vi "Path_to_Array_Of_Filepaths.vi"(4 "length":i32=1, 6 "offset (for subset of folder)":i32, 8 "error in (no error)":errorcluster, 11 "File or Folder Path":path=path "C:/") -> (0 "error out":errorcluster, 1 "pattern":string="*.dat", 3 "array of files":path[](array[path]))   [LabVIEW 2016]
uses:
  <userlib>/LevyLab/LV to ITX/LVtoITX.lvclass
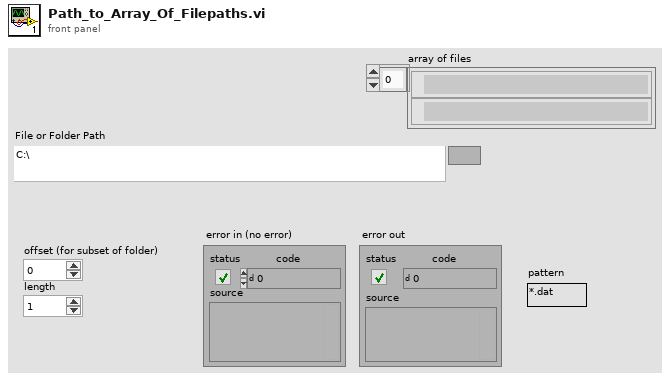
[diagram p1: front panel]
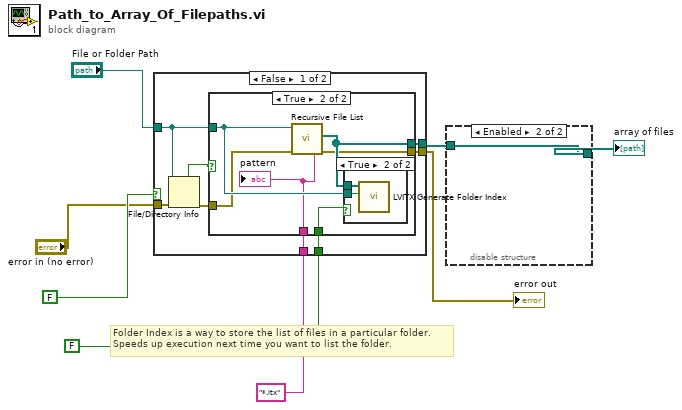
[diagram p0: block diagram]
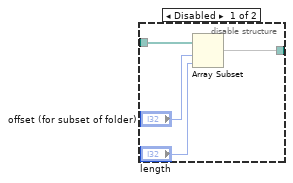
[diagram p2: hidden frame]
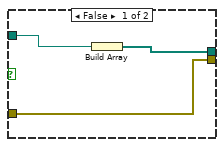
[diagram p3: hidden frame]
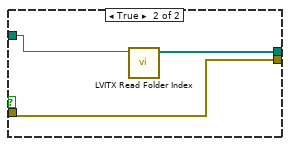
[diagram p5: hidden frame]
diagram:
  # "Folder Index is a way to store the list of files in a particular folder.\nSpeeds up execution next time you want to list the folder."
  n1 = case shown="False" FALSE ("Use Folder Index File?") {
    tunnel: [w14 w29] -> w5
    tunnel: "File or Folder Path" -> [w16 w30]
    tunnel: FALSE ("Generate Folder Index File?") -> [w13 _]
    tunnel: "*.itx" ("pattern") -> [w12 _]
    tunnel: "error in (no error)" -> [w11 w28]
    tunnel: [w9 w28] -> w1
    frame False {
      n2 = File/Directory Info(path=w16, error in=w11) -> (directory=w15:bool, error out=w10:errorcluster)  [unwired: 5 out]
      n3 = case shown="True" w15 {
        tunnel: [w19 w23] -> w14
        tunnel: w16 -> [w18 w25]
        tunnel: w13 -> [_ w24]
        tunnel: w12 -> [_ w22]
        tunnel: w10 -> [w17 w21]
        tunnel: [w17 w20] -> w9
        frame False {
          n4 = Build Array(w18) -> (w19:path[])
        }
        frame True {
          n5 = call <vilib>:"Recursive File List.vi"("pattern"=w22, "error in (no error)"=w21, "Folder Path"=w25) -> ("error out"=w20:errorcluster, "All Files in Dir"=w23:path[])  [unwired: 4 in, 3 out]
          n6 = case shown="True" w24 {
            tunnel: w23 -> [_ w27]
            tunnel: w25 -> [_ w26]
            frame False {
            }
            frame True {
              n7 = call <userlib>:"LVITX Generate Folder Index.vi"("File or Folder Path"=w26, "All Files in Dir"=w27) -> ()  [unwired: 10 in]
            }
          }
          "pattern" <- w22
        }
      }
    }
    frame True {
      n8 = call <userlib>:"LVITX Read Folder Index.vi"("File or Folder Path"=w30) -> ("Array"=w29:path[])  [unwired: 10 in]
    }
  }
  "error out" <- w1
  n9 = disable-structure shown="Enabled" {
    disable-tunnel: [w34 w35] -> w8
    disable-tunnel: w5 -> [w31 w35]
    frame Disabled {
      n10 = Array Subset(array=w31, index="offset (for subset of folder)", length="length") -> (w34:path[])
    }
    frame Enabled {
    }
  }
  "array of files" <- w8
